vi "引导界面.vi"   [LabVIEW 2020]
types:
  T1 = enum32{"Invalid", "Standard", "Closed", "Hidden", "Minimized", "Maximized"}
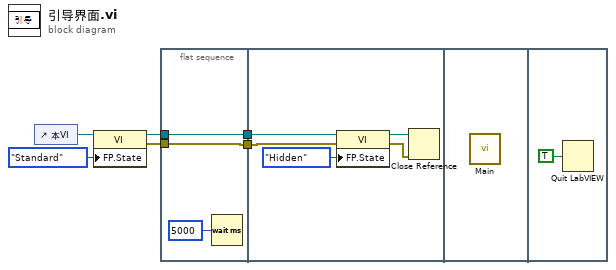
[diagram p0: block diagram]
diagram:
  n1 = control-ref of="本VI"() -> (w5:refnum<vi>)
  n2 = property class="VI"(reference=w5, "FP.State"=T1."Standard" ("前面板窗口:状态")) -> (reference out=w4:refnum<vi>, error out=w2:errorcluster)  [unwired: 1 in]
  n3 = flat-sequence {
    tunnel: w4 -> [w8]
    tunnel: [w8] -> w3
    tunnel: w2 -> [w7]
    tunnel: [w7] -> w1
    tunnel: w3 -> [w11]
    tunnel: w1 -> [w10]
    frame #0 {
      n4 = Wait (ms)(milliseconds to wait=u32 5000 ("等待时间（毫秒）")) -> ()  [unwired: 1 out]
    }
    frame #1 {
      n5 = property class="VI"(reference=w11, error in=w10, "FP.State"=T1."Hidden" ("前面板窗口:状态")) -> (reference out=w14:refnum<vi>, error out=w13:errorcluster)
      n6 = Close Reference(reference=w14, error in (no error)=w13) -> ()  [unwired: 1 out]
    }
    frame #2 {
      n7 = call "Main.vi"() -> ()  [unwired: 12 in]
    }
    frame #3 {
      n8 = Quit LabVIEW(quit? (T)=TRUE ("退出？(T)")) -> ()
    }
  }
